vi "TCL INIT.vi"   [LabVIEW 2009]
uses:
  TCL Global.vi
  <vilib>/Utility/config.llb/Read Key (String).vi
  <vilib>/Utility/config.llb/Read Key (Path).vi
  TPS Global.vi
  <vilib>/Utility/config.llb/NI_LVConfig.lvlib
types:
  T1 = typedef "NI_LVConfig.lvlib/Config Data RefNum.ctl" = refnum<k1>
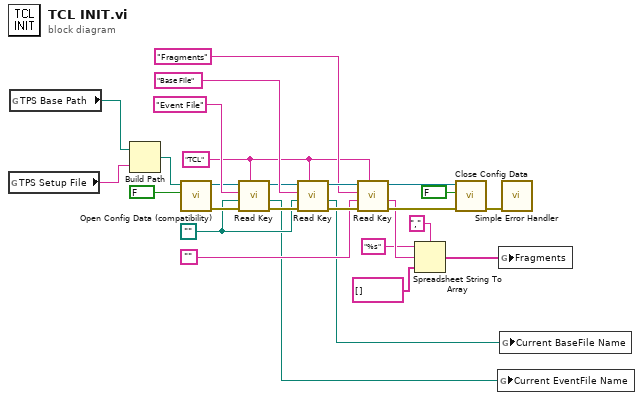
[diagram p0: block diagram]
diagram:
  w4 = path ""
  w12 = "TCL" ("section")
  n1 = global read "TPS Global.vi" "TPS Setup File"() -> (w27:string)
  n2 = global read "TPS Global.vi" "TPS Base Path"() -> (w6:path)
  n3 = Build Path(base path=w6, name or relative path=w27) -> (appended path=w22:path)
  n4 = call <vilib>:"Open Config Data (compatibility).vi"("create file if necessary (T)"=FALSE ("create file if necessary? (T)"), "configuration file path"=w22) -> ("error out"=w24:errorcluster, "refnum"=w25:T1)  [unwired: 7 in, 1 out]
  n5 = call-poly <vilib>:"Read Key.vi"("section"=w12, "error in (no error)"=w24, "default value"=w4, "key"="Event File", "refnum"=w25) -> ("error out"=w20:errorcluster, "value"=w2:path, "refnum out"=w19:T1)  [unwired: 3 in, 1 out]
  n6 = call-poly <vilib>:"Read Key.vi"("section"=w12, "error in (no error)"=w20, "default value"=w4, "key"="Base File", "refnum"=w19) -> ("error out"=w17:errorcluster, "value"=w3:path, "refnum out"=w15:T1)  [unwired: 3 in, 1 out]
  n7 = call-poly <vilib>:"Read Key.vi"("section"=w12, "error in (no error)"=w17, "default value"="", "key"="Fragments", "refnum"=w15) -> ("error out"=w16:errorcluster, "value"=w11:string, "refnum out"=w14:T1)  [unwired: 3 in, 1 out]
  n8 = Spreadsheet String To Array(delimiter (Tab)=",", format string="%s", spreadsheet string=w11, array type (2D Dbl)=string[] [] ("Array Constant")) -> (array=w7:string[])
  n9 = call <vilib>:"Close Config Data.vi"("error in (no error)"=w16, "write file if changed (T)"=FALSE, "refnum"=w14) -> ("error out"=w18:errorcluster)  [unwired: 7 in, 1 out]
  n10 = global write "TCL Global.vi" "Current EventFile Name"(w2) -> ()
  n11 = global write "TCL Global.vi" "Fragments"(w7) -> ()
  n12 = global write "TCL Global.vi" "Current BaseFile Name"(w3) -> ()
  n13 = call <vilib>:"Simple Error Handler.vi"("error in (no error)"=w18) -> ()  [unwired: 4 in, 5 out]
